vi "Random Competition.vi"() -> ()   [LabVIEW 2021]
panel:
  out "A vs B":cluster{i32[], i32[]}(graph)
  out "Tie":bool
  out "Winner B":bool
  out "Winner A":bool
  out "Points B":i32
  out "Points A":i32
  out "Random Number B":dbl
  out "Random Number A":dbl
  in  "Number of Iterations":i32
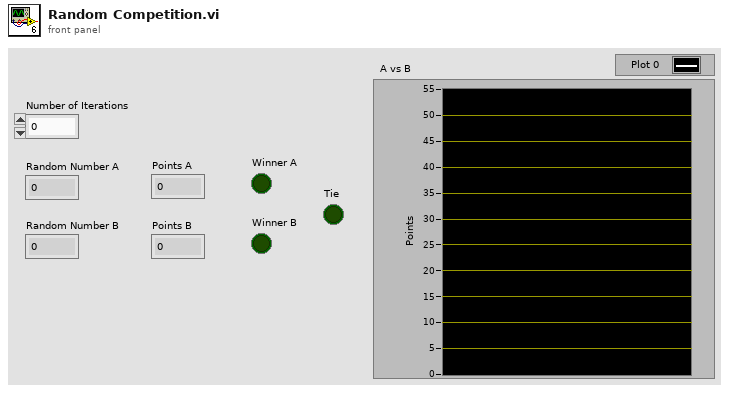
[diagram p1: front panel]
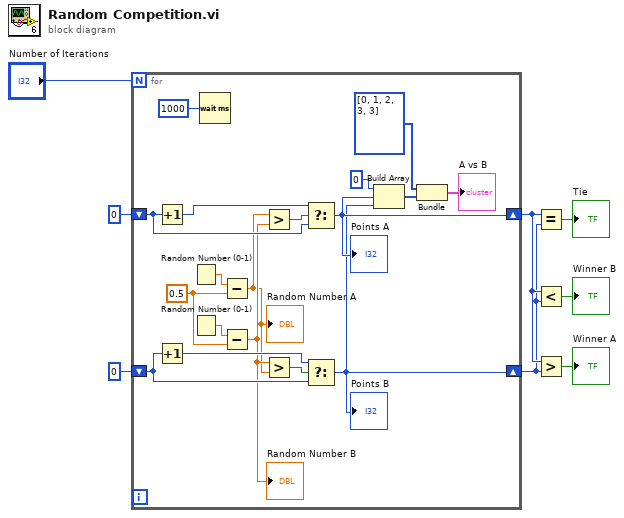
[diagram p0: block diagram]
diagram:
  n1 = for {
    N: "Number of Iterations" -> [_]
    shift-right: [w12] -> w6
    shift-left: 0 -> [w20]
    shift-right: [w11] -> w5
    shift-left: 0 -> [w22]
    w24 = 0.5
    n2 = Increment(x=w20) -> (x+1=w21:i32)
    n3 = Increment(x=w22) -> (x+1=w23:i32)
    n4 = Random Number (0-1)() -> (number: 0 to 1=w26:dbl)
    n5 = Random Number (0-1)() -> (number: 0 to 1=w25:dbl)
    n6 = Wait (ms)(milliseconds to wait=1000) -> ()  [unwired: 1 out]
    n7 = Subtract(x=w26, y=w24) -> (x-y=w17:dbl)
    "Random Number A" <- w17
    n8 = Subtract(x=w25, y=w24) -> (x-y=w18:dbl)
    "Random Number B" <- w18
    n9 = Greater?(x=w17, y=w18) -> (0:w19:bool)
    n10 = Greater?(x=w18, y=w17) -> (0:w16:bool)
    n11 = Select(t=w21, s=w19, f=w20) -> (s? t:f=w12:i32)
    "Points A" <- w12
    n12 = Select(t=w23, s=w16, f=w22) -> (s? t:f=w11:i32)
    "Points B" <- w11
    n13 = Build Array(0, w12, w11) -> (w10:i32[])
    n14 = Bundle(i32[] [0, 1, 2, 3, 3], w10) -> (→"A vs B":cluster{i32[], i32[]})  [unwired: 1 in]
  }
  n15 = Equal?(x=w6, y=w5) -> (x = y?=→"Tie":bool)
  n16 = Less?(x=w6, y=w5) -> (x < y?=→"Winner B":bool)
  n17 = Greater?(x=w6, y=w5) -> (0:→"Winner A":bool)
